vi "slam_ortogonal_(x,y).versao3.vi"() -> ()   [LabVIEW 2016]
uses:
  <vilib>/NXT/Subs/LVHSConnector.ctl
  <vilib>/NXT/LegoClasses/BrickReference/BrickReference.lvclass
  <vilib>/NXT/Block Support/NXT_OutputPort.ctl
  <vilib>/NXT/NXTIO Xnodes/NXTIONodeSubVIs/NXTStopMotors.vi
  <vilib>/NXT/NXTIO Xnodes/NXTIONodeSubVIs/NXTMoveMotors.vi
  <vilib>/NXT/Dual Mode Library/Waits/Wait_Num.vi
  <vilib>/NXT/NXTIO Xnodes/AddressXNode/NXTIOAddress.xnode
  <vilib>/NXT/NXTIO Xnodes/NXTIOXNode/NXTIO.xnode
panel:
  out "yo":dbl format="%#_13g"
  out "dx":dbl format="%#_13g"
  out "dy":dbl format="%#_13g"
  out "xo":dbl format="%#_13g"
  out "NXT/EV3 2":T1
  in  "NXT/EV3":T1
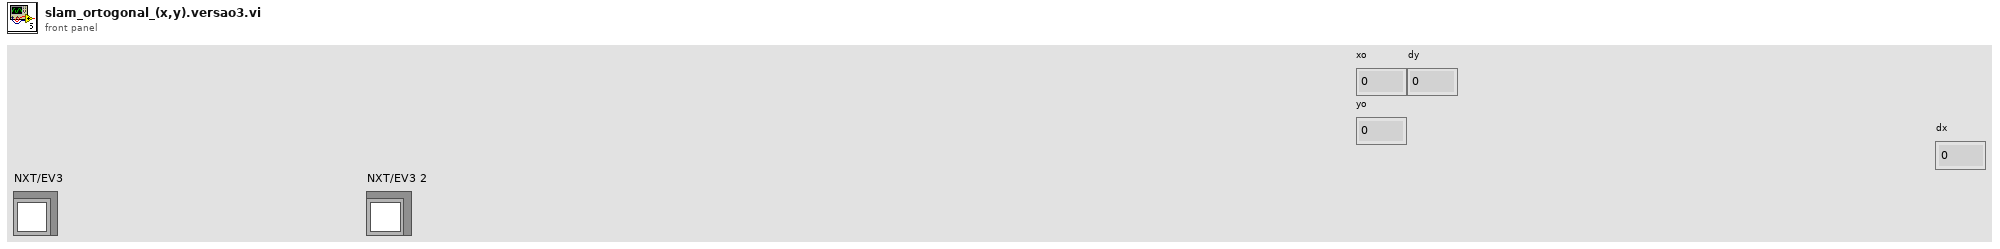
[diagram p1: front panel]
types:
  T1 = typedef "LVHSConnector.ctl" = refnum<class "BrickReference.lvclass">
  T2 = typedef "NXT_OutputPort.ctl" = u8
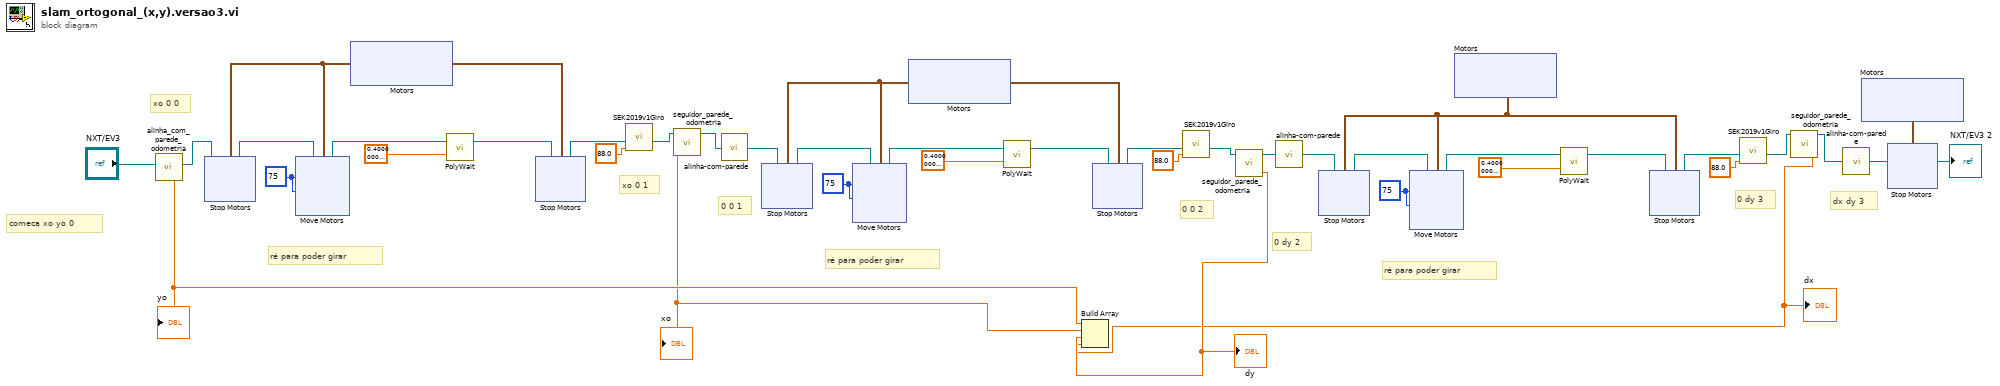
[diagram p0: block diagram]
diagram:
  w16 = i8 75 ("Power/Speed 1")
  w27 = i8 75 ("Power/Speed 1")
  w36 = i8 75 ("Power/Speed 1")
  # "dx dy 3"
  # "0 dy 3"
  # "ré para poder girar"
  # "0 dy 2"
  # "0 0 2"
  # "ré para poder girar"
  # "0 0 1"
  # "xo 0 1"
  # "ré para poder girar"
  # "xo 0 0"
  # "comeca xo yo 0"
  n1 = call "alinha_com_parede_odometria.vi"("NXT/EV3"="NXT/EV3") -> ("Numeric"=w4:dbl, "NXT/EV3 2"=w9:T1)  [unwired: 9 in]
  "yo" <- w4
  n2 = xnode "Motors"() -> ("Motor"=w32:cluster{"Port":T2, "Port":T2})
  n3 = xnode "Stop Motors"("Motors"=w32, "NXT/EV3"=w9) -> ("NXT/EV3"=w37:T1)
  n4 = xnode "Move Motors"("Power/Speed 2"=w36, "Power/Speed 1"=w36, "Motors"=w32, "NXT/EV3"=w37) -> ("NXT/EV3"=w38:T1)
  n5 = call-poly <vilib>:"PolyWait.vi"("Time (1 sec)"=sgl 0.4, "NXT/EV3"=w38) -> ("NXT/EV3"=w40:T1)  [unwired: 2 in]
  n6 = xnode "Stop Motors"("Motors"=w32, "NXT/EV3"=w40) -> ("NXT/EV3"=w35:T1)
  n7 = call "SEK2019v1Giro.vi"("ANGULO"=sgl 88.0, "NXT/EV3"=w35) -> ("NXT/EV3 2"=w33:T1)  [unwired: 9 in]
  n8 = call "seguidor_parede_odometria.vi"("NXT/EV3 3"=w33) -> ("Numeric"=w3:dbl, "NXT/EV3 2"=w31:T1)  [unwired: 3 in]
  "xo" <- w3
  n9 = call "alinha-com-parede.vi"("NXT/EV3"=w31) -> ("NXT/EV3 2"=w22:T1)  [unwired: 4 in]
  n10 = xnode "Motors"() -> ("Motor"=w30:cluster{"Port":T2, "Port":T2})
  n11 = xnode "Stop Motors"("Motors"=w30, "NXT/EV3"=w22) -> ("NXT/EV3"=w26:T1)
  n12 = xnode "Move Motors"("Power/Speed 2"=w27, "Power/Speed 1"=w27, "Motors"=w30, "NXT/EV3"=w26) -> ("NXT/EV3"=w25:T1)
  n13 = call-poly <vilib>:"PolyWait.vi"("Time (1 sec)"=sgl 0.4, "NXT/EV3"=w25) -> ("NXT/EV3"=w23:T1)  [unwired: 2 in]
  n14 = xnode "Stop Motors"("Motors"=w30, "NXT/EV3"=w23) -> ("NXT/EV3"=w28:T1)
  n15 = call "SEK2019v1Giro.vi"("ANGULO"=sgl 88.0, "NXT/EV3"=w28) -> ("NXT/EV3 2"=w8:T1)  [unwired: 9 in]
  n16 = call "seguidor_parede_odometria.vi"("NXT/EV3 3"=w8) -> ("Numeric"=w2:dbl, "NXT/EV3 2"=w7:T1)  [unwired: 3 in]
  "dy" <- w2
  n17 = call "alinha-com-parede.vi"("NXT/EV3"=w7) -> ("NXT/EV3 2"=w21:T1)  [unwired: 4 in]
  n18 = xnode "Motors"() -> ("Motor"=w10:cluster{"Port":T2, "Port":T2})
  n19 = xnode "Stop Motors"("Motors"=w10, "NXT/EV3"=w21) -> ("NXT/EV3"=w17:T1)
  n20 = xnode "Move Motors"("Power/Speed 2"=w16, "Power/Speed 1"=w16, "Motors"=w10, "NXT/EV3"=w17) -> ("NXT/EV3"=w18:T1)
  n21 = call-poly <vilib>:"PolyWait.vi"("Time (1 sec)"=sgl 0.4, "NXT/EV3"=w18) -> ("NXT/EV3"=w20:T1)  [unwired: 2 in]
  n22 = xnode "Stop Motors"("Motors"=w10, "NXT/EV3"=w20) -> ("NXT/EV3"=w15:T1)
  n23 = call "SEK2019v1Giro.vi"("ANGULO"=sgl 88.0, "NXT/EV3"=w15) -> ("NXT/EV3 2"=w6:T1)  [unwired: 9 in]
  n24 = call "seguidor_parede_odometria.vi"("NXT/EV3 3"=w6) -> ("Numeric"=w1:dbl, "NXT/EV3 2"=w5:T1)  [unwired: 3 in]
  "dx" <- w1
  n25 = Build Array(w4, w3, w2, w1) -> ()  [unwired: 1 out]
  n26 = call "alinha-com-parede.vi"("NXT/EV3"=w5) -> ("NXT/EV3 2"=w12:T1)  [unwired: 4 in]
  n27 = xnode "Motors"() -> ("Motor"=w13:cluster{"Port":T2, "Port":T2})
  n28 = xnode "Stop Motors"("Motors"=w13, "NXT/EV3"=w12) -> ("NXT/EV3"=→"NXT/EV3 2":T1)
